vi "Create APU Listbox IP Text.vi"(8 "error in (no error)":errorcluster, 10 "ips available":string[](array[string]), 11 "Section Ref in":T1 format="%.0x") -> (0 "error out":errorcluster, 2 "listbox text":string[][](array[string]), 3 "Section Ref out":T1 format="%.0x", 5 "not present item indexes":i32[](array[numeric]))   [LabVIEW 2015, in "Engine Simulation Toolkit System Explorer.lvlib"]
uses:
  Engine Simulation Toolkit System Explorer.lvlib
  <vilib>/NI Veristand/Custom Device API/Custom Device Item Ref.ctl
  Shared/Properties.vi
  <vilib>/NI Veristand/Custom Device API/Get Item Property (String).vi
  Shared/Constants and GUIDs.vi
  <vilib>/NI Veristand/Custom Device API/Custom Device API.lvlib
  Shared/Engine Simulation Toolkit Shared.lvlib
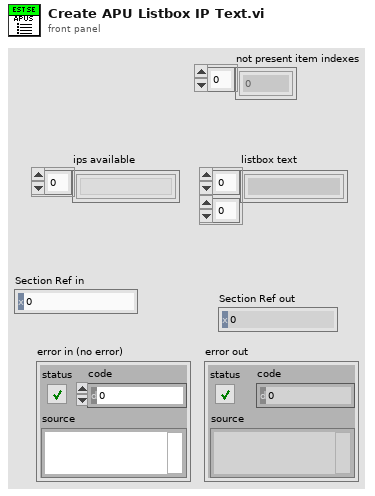
[diagram p1: front panel]
types:
  T1 = typedef "Custom Device API.lvlib/Custom Device Item Ref.ctl" = u64
  T2 = typedef "Custom Device API.lvlib/Custom Device Item Info.ctl" = cluster{"Name":string, "Is Channel":bool, "GUID":string, "Is Waveform":bool}
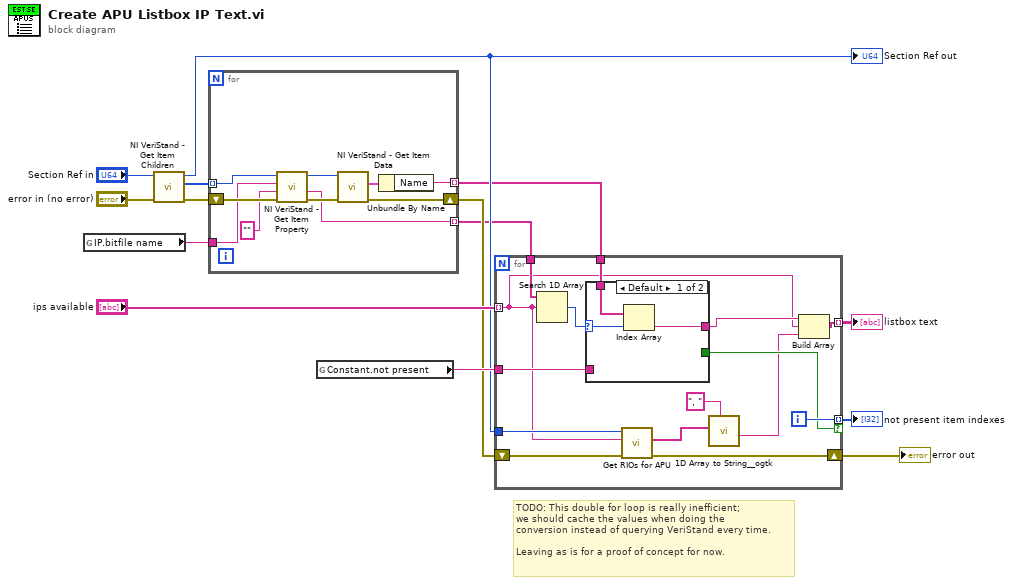
[diagram p0: block diagram]
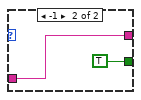
[diagram p2: hidden frame]
diagram:
  # "TODO: This double for loop is really inefficient;\nwe should cache the values when doing the\nconversion instead of querying VeriStand every time.\n\nLeaving as is for a proof of concept for now."
  n1 = global read "Properties.vi" "IP.bitfile name"() -> (w10:string)
  n2 = call <vilib>:"NI VeriStand - Get Item Children.vi"("error in (no error)"="error in (no error)", "Item Ref in"="Section Ref in") -> ("error out"=w12:errorcluster, "Child Refs"=w11:T1[], "Item Ref out"=w4:T1)  [unwired: 6 in, 1 out]
  "Section Ref out" <- w4
  n3 = for {
    shift-right: [w19] -> w5
    shift-left: w12 -> [w24]
    tunnel: w11 -> [w22] mode=indexing
    tunnel: w10 -> [w21]
    tunnel: [w16] -> w3 mode=indexing
    tunnel: [w15] -> w2 mode=indexing
    n4 = call-poly <vilib>:"NI VeriStand - Get Item Property.vi"("error in (no error)"=w24, "Default Value"="", "Property Name"=w21, "Item Ref in"=w22) -> ("error out"=w23:errorcluster, "Value"=w16:string, "Item Ref out"=w18:T1)  [unwired: 4 in, 1 out]
    n5 = call <vilib>:"NI VeriStand - Get Item Data.vi"("error in (no error)"=w23, "Item Ref in"=w18) -> ("error out"=w19:errorcluster, "Item Info"=w17:T2)  [unwired: 6 in, 2 out]
    n6 = Unbundle By Name(w17) -> ("Name"=w15:string)
  }
  n7 = global read "Constants and GUIDs.vi" "Constant.not present"() -> (w7:string)
  n8 = for {
    tunnel: "ips available" -> [w25] mode=indexing
    tunnel: w3 -> [w32]
    tunnel: w2 -> [w38]
    tunnel: [w36] -> w8 mode=indexing
    tunnel: w7 -> [w35]
    tunnel: [w34] -> w6 mode=indexing if=w33
    shift-right: [w29] -> w1
    shift-left: w5 -> [w28]
    tunnel: w4 -> [w27]
    i -> [w34]
    n9 = Search 1D Array(1D array=w32, element=w25) -> (index of element=w39:i32)  [unwired: 1 in]
    n10 = case shown="Default" w39 {
      selector: w39 -> [w41 _]
      tunnel: [w40 w44] -> w37
      tunnel: w38 -> [w42 _]
      tunnel: w35 -> [_ w44]
      tunnel: [_ TRUE] -> w33
      frame Default {
        n11 = Index Array(array=w42, index=w41) -> (element=w40:string)
      }
      frame -1 {
      }
    }
    n12 = call "Get RIOs for APU.vi"("error in (no error)"=w28, "APU name"=w25, "Item Ref in"=w27) -> ("error out"=w29:errorcluster, "RIO Addresses"=w26:string[])  [unwired: 6 in, 1 out]
    n13 = call <userlib>:"1D Array to String__ogtk.vi"("delimiter (Tab)"=", ", "Array of Strings"=w26) -> ("delimited string"=w30:string)  [unwired: 9 in]
    n14 = Build Array(w37, w25, w30) -> (w36:string[])
  }
  "error out" <- w1
  "listbox text" <- w8
  "not present item indexes" <- w6
